vi "Write Digital Port.vi"(8 "error in (no error)":errorcluster, 10 "Relay Mode":bool[](array[boolean]), 11 "NI 6514 in":refnum<class "NI 6514.lvclass">) -> (0 "error out":errorcluster, 3 "NI 6514 out":refnum<class "NI 6514.lvclass">)   [LabVIEW 2019, in "Concrete.lvlib" / "NI 6514.lvclass"]
uses:
  NI 6514.lvclass
  NI 6514.lvclass/NI 6514.ctl
  <vilib>/DAQmx/write.llb/DAQmx Write (Digital 1D Bool 1Chan 1Samp).vi
  <vilib>/DAQmx/miscellaneous.llb/DAQmx Fill In Error Info.vi
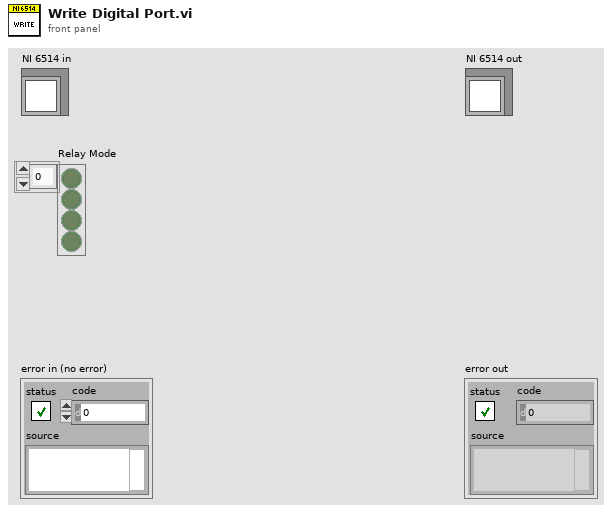
[diagram p1: front panel]
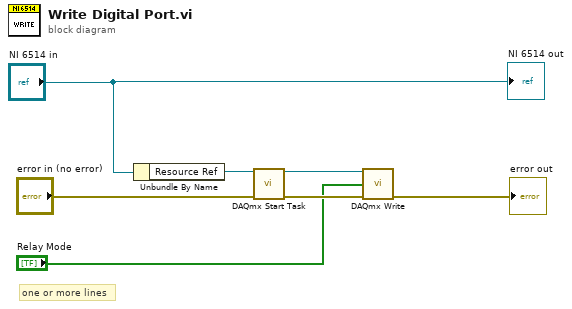
[diagram p0: block diagram]
diagram:
  # "one or more lines"
  n1 = Unbundle By Name("NI 6514 in") -> ("Resource Ref"=w3:refnum<k21>)
  n2 = call <vilib>:"DAQmx Start Task.vi"("task/channels in"=w3, "error in"="error in (no error)") -> ("task out"=w2:refnum<k21>, "error out"=w7:errorcluster)  [unwired: 12 in]
  n3 = call-poly <vilib>:"DAQmx Write.vi"("task/channels in"=w2, "data"="Relay Mode", "error in"=w7) -> ("error out"=→"error out":errorcluster)  [unwired: 10 in, 2 out]
  "NI 6514 out" <- "NI 6514 in"
